vi "putNodeInOpen.vi"(8 "error in (no error)":errorcluster, 9 "SearchMethod":T1, 10 "MultiTreeNode":refnum<data-value>, 11 "MultiTree in":refnum<class "MultiTree.lvclass">) -> (0 "error out":errorcluster, 3 "MultiTree out":refnum<class "MultiTree.lvclass">)   [LabVIEW 2014, in "MultiTree.lvlib" / "MultiTree.lvclass"]
uses:
  <userlib>/AdvancedDataStructures/ClassBased/MultiTree/MultiTree.lvclass
  <userlib>/AdvancedDataStructures/ClassBased/MultiTree/SearchMethod.ctl
  <userlib>/AdvancedDataStructures/ClassBased/MultiTreeNode/MultiTreeNode.lvclass
  <userlib>/AdvancedDataStructures/ClassBased/MultiTree/MultiTree.lvclass/MultiTree.ctl
  <userlib>/AdvancedDataStructures/ClassBased/LinkedList/position.ctl
  <userlib>/AdvancedDataStructures/ClassBased/MultiTreeNode/MultiTreeNode.lvclass/MultiTreeNode.ctl
  <userlib>/AdvancedDataStructures/ClassBased/LinkedList/InsertSearchOptions.ctl
  <userlib>/AdvancedDataStructures/ClassBased/LinkedList/LinkedList.lvclass
  <userlib>/AdvancedDataStructures/ClassBased/Common/BasicSortedList/BasicSortedList/BasicSortedList.lvclass
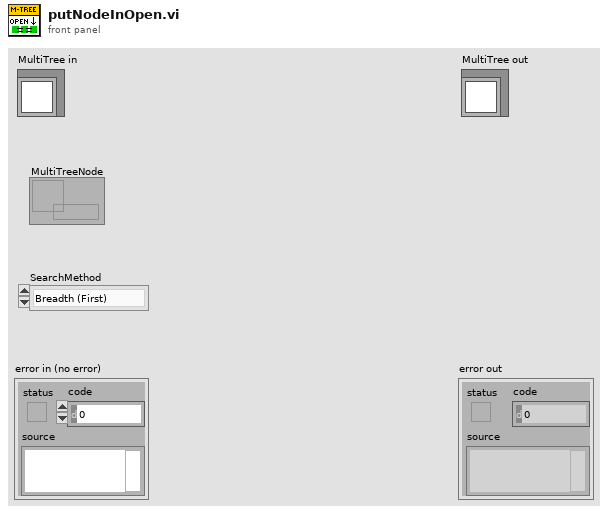
[diagram p1: front panel]
types:
  T1 = typedef "MultiTree.lvlib/MultiTree.lvclass/SearchMethod.ctl" = enum16{"Breadth (First)", "Depth (First)", "Best First", "Breadth (Exhaustive)", "Depth (Exhaustive)"}
  T2 = typedef "LinkedList.lvlib/LinkedList.lvclass/position.ctl" = enum16{"Front", "Back", "Search"}
  T3 = typedef "LinkedList.lvlib/LinkedList.lvclass/InsertSearchOptions.ctl" = cluster{"InsertIfEmpty":bool, "Insert After":bool, "InsertIfNotFound":bool}
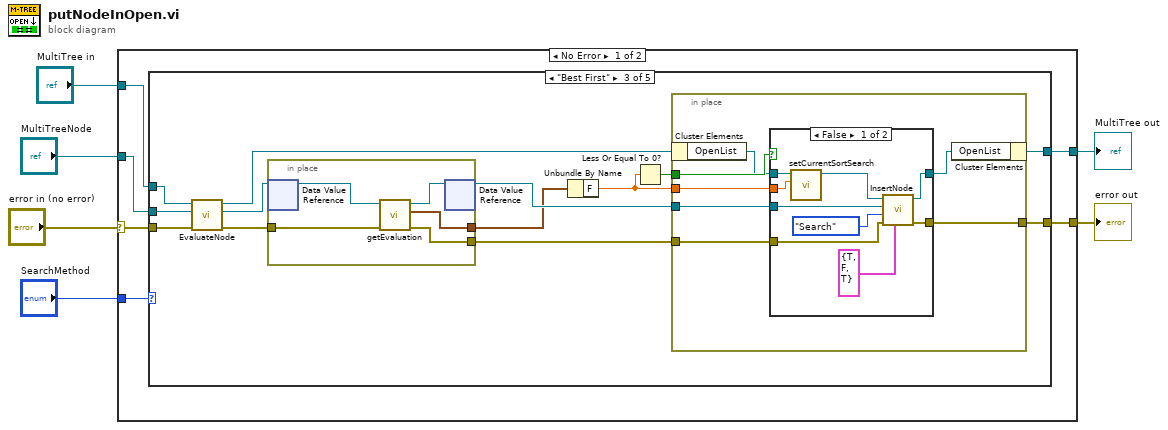
[diagram p0: block diagram]
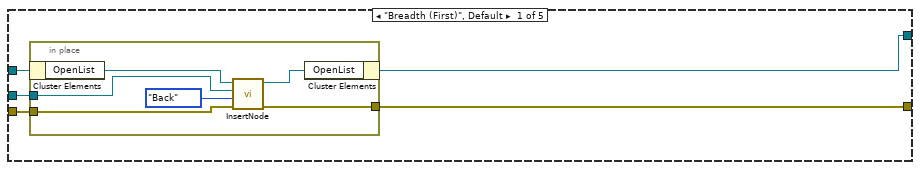
[diagram p2: hidden frame]
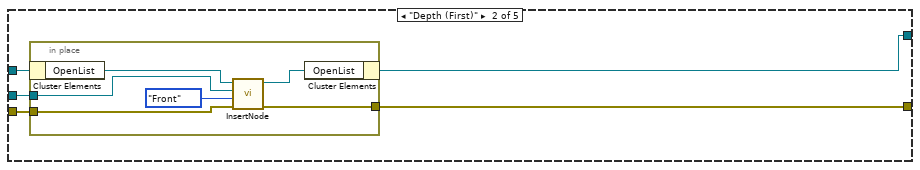
[diagram p3: hidden frame]
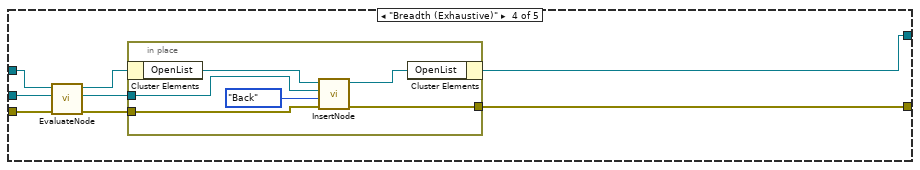
[diagram p5: hidden frame]
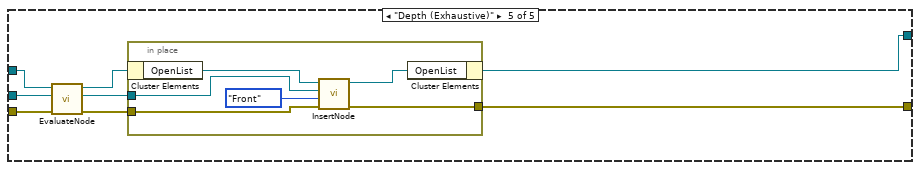
[diagram p6: hidden frame]
diagram:
  n1 = case shown="No Error" "error in (no error)" {
    selector: "error in (no error)" -> [w8 w100]
    tunnel: [w7 w100] -> w5
    tunnel: [w11 w99] -> w3
    tunnel: "MultiTree in" -> [w12 w99]
    tunnel: "SearchMethod" -> [w10 _]
    tunnel: "MultiTreeNode" -> [w9 _]
    frame No Error {
      n2 = case shown="\"Best First\"" w10 {
        tunnel: w9 -> [w17 w28 w42 w76 w86]
        tunnel: w8 -> [w16 w27 w41 w77 w87]
        tunnel: [w15 w26 w46 w71 w85] -> w7
        tunnel: w12 -> [w14 w25 w43 w78 w89]
        tunnel: [w13 w24 w37 w74 w88] -> w11
        frame "Breadth (First)", Default {
          n3 = in-place {
            in-place-border: w17 -> [w23]
            in-place-border: w16 -> [w22]
            in-place-border: [w20] -> w15
            n4 = in-place-cluster #1(w14) -> ("OpenList"=w19:refnum<class "BasicSortedList.lvclass">)
            n5 = call <userlib>:"InsertNode.vi"("error in (no error)"=w22, "position"=position."Back", "ToInsert"=w23, "LinkedList in"=w19) -> ("error out"=w20:errorcluster, "LinkedList out"=w18:refnum<class "BasicSortedList.lvclass">)  [unwired: 5 in, 1 out]
            n6 = in-place-cluster #1("OpenList"=w18) -> (w13:refnum<class "MultiTree.lvclass">)
          }
        }
        frame "Depth (First)" {
          n7 = in-place {
            in-place-border: w28 -> [w33]
            in-place-border: w27 -> [w32]
            in-place-border: [w31] -> w26
            n8 = in-place-cluster #2(w25) -> ("OpenList"=w30:refnum<class "BasicSortedList.lvclass">)
            n9 = call <userlib>:"InsertNode.vi"("error in (no error)"=w32, "position"=position."Front", "ToInsert"=w33, "LinkedList in"=w30) -> ("error out"=w31:errorcluster, "LinkedList out"=w29:refnum<class "BasicSortedList.lvclass">)  [unwired: 5 in, 1 out]
            n10 = in-place-cluster #2("OpenList"=w29) -> (w24:refnum<class "MultiTree.lvclass">)
          }
        }
        frame "Best First" {
          n11 = call <userlib>:"EvaluateNode.vi"("error in (no error)"=w41, "ToEvaluate in"=w42, "MultiTree in"=w43) -> ("error out"=w39:errorcluster, "ToEvaluate out"=w40:refnum<data-value>, "MultiTree out"=w38:refnum<class "MultiTree.lvclass">)  [unwired: 6 in]
          n12 = in-place {
            in-place-border: [w68] -> w47
            in-place-border: w39 -> [w69]
            in-place-border: [w67] -> w36
            n13 = in-place-dvr #3(w40) -> (w70:refnum<class "MultiTreeNode.lvclass">)  [unwired: 1 out]
            n14 = call <userlib>:"getEvaluation.vi"("error in (no error)"=w69, "MultiTreeNode in"=w70) -> ("error out"=w68:errorcluster, "evaluation"=w67:cluster{"F":dbl, "G":dbl, "H":dbl}, "MultiTreeNode out"=w66:refnum<class "MultiTreeNode.lvclass">)  [unwired: 7 in]
            n15 = in-place-dvr #3(w66) -> (w45:refnum<data-value>)  [unwired: 1 out]
          }
          n16 = Unbundle By Name(w36) -> ("F"=w35:dbl)
          n17 = Less Or Equal To 0?(x=w35) -> (x <= 0?=w44:bool)
          n18 = in-place {
            in-place-border: w47 -> [w54]
            in-place-border: [w53] -> w46
            in-place-border: w45 -> [w52]
            in-place-border: w35 -> [w51]
            in-place-border: w44 -> [w50]
            n19 = in-place-cluster #4(w38) -> ("OpenList"=w49:refnum<class "BasicSortedList.lvclass">)
            n20 = case shown="False" w50 {
              tunnel: w49 -> [w57 w65]
              tunnel: [w63 w65] -> w48
              tunnel: w54 -> [w58 w64]
              tunnel: [w61 w64] -> w53
              tunnel: w52 -> [w60 _]
              tunnel: w51 -> [w55 _]
              frame False {
                n21 = call <userlib>:"setCurrentSortSearch.vi"("CurrentSortSearch"=w55, "BasicSortedList in"=w57) -> ("BasicSortedList out"=w56:refnum<class "BasicSortedList.lvclass">)  [unwired: 8 in, 1 out]
                n22 = call <userlib>:"InsertNode.vi"("Insert Search"=T3 {"InsertIfEmpty"=TRUE, "Insert After"=FALSE, "InsertIfNotFound"=TRUE}, "error in (no error)"=w58, "position"=position."Search", "ToInsert"=w60, "LinkedList in"=w56) -> ("error out"=w61:errorcluster, "LinkedList out"=w63:refnum<class "BasicSortedList.lvclass">)  [unwired: 4 in, 1 out]
              }
              frame True {
              }
            }
            n23 = in-place-cluster #4("OpenList"=w48) -> (w37:refnum<class "MultiTree.lvclass">)
          }
        }
        frame "Breadth (Exhaustive)" {
          n24 = call <userlib>:"EvaluateNode.vi"("error in (no error)"=w77, "ToEvaluate in"=w76, "MultiTree in"=w78) -> ("error out"=w72:errorcluster, "ToEvaluate out"=w73:refnum<data-value>, "MultiTree out"=w75:refnum<class "MultiTree.lvclass">)  [unwired: 6 in]
          n25 = in-place {
            in-place-border: w73 -> [w84]
            in-place-border: w72 -> [w79]
            in-place-border: [w82] -> w71
            n26 = in-place-cluster #5(w75) -> ("OpenList"=w81:refnum<class "BasicSortedList.lvclass">)
            n27 = call <userlib>:"InsertNode.vi"("error in (no error)"=w79, "position"=position."Back", "ToInsert"=w84, "LinkedList in"=w81) -> ("error out"=w82:errorcluster, "LinkedList out"=w80:refnum<class "BasicSortedList.lvclass">)  [unwired: 5 in, 1 out]
            n28 = in-place-cluster #5("OpenList"=w80) -> (w74:refnum<class "MultiTree.lvclass">)
          }
        }
        frame "Depth (Exhaustive)" {
          n29 = call <userlib>:"EvaluateNode.vi"("error in (no error)"=w87, "ToEvaluate in"=w86, "MultiTree in"=w89) -> ("error out"=w90:errorcluster, "ToEvaluate out"=w91:refnum<data-value>, "MultiTree out"=w92:refnum<class "MultiTree.lvclass">)  [unwired: 6 in]
          n30 = in-place {
            in-place-border: w91 -> [w98]
            in-place-border: w90 -> [w93]
            in-place-border: [w96] -> w85
            n31 = in-place-cluster #6(w92) -> ("OpenList"=w95:refnum<class "BasicSortedList.lvclass">)
            n32 = call <userlib>:"InsertNode.vi"("error in (no error)"=w93, "position"=position."Front", "ToInsert"=w98, "LinkedList in"=w95) -> ("error out"=w96:errorcluster, "LinkedList out"=w94:refnum<class "BasicSortedList.lvclass">)  [unwired: 5 in, 1 out]
            n33 = in-place-cluster #6("OpenList"=w94) -> (w88:refnum<class "MultiTree.lvclass">)
          }
        }
      }
    }
    frame Error {
    }
  }
  "error out" <- w5
  "MultiTree out" <- w3
